vi "Realsense Cam Config Stream.vi"(8 "error in (no error)":errorcluster, 10 "Streams":T1[](array[typedef]), 11 "Realsense Cam in":refnum<class "Realsense Cam.lvclass">) -> (0 "error out":errorcluster, 3 "Realsense Cam out":refnum<class "Realsense Cam.lvclass">)   [LabVIEW 2018, in "Realsense Cam.lvclass"]
uses:
  Realsense Cam.lvclass
  Private/Stream Types Enum STYP.ctl
  Realsense Cam.lvclass/Realsense Cam.ctl
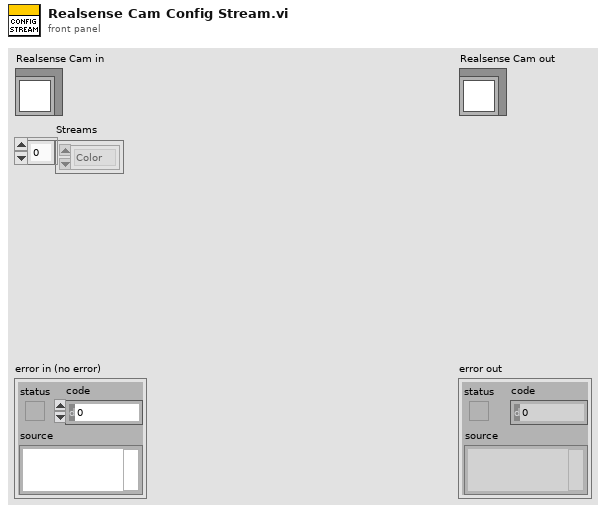
[diagram p1: front panel]
types:
  T1 = typedef "Realsense Cam.lvclass/Stream Types Enum STYP.ctl" = enum16{"Depth", "Left IR", "Right IR", "Color", "RGB Ext.", "Left IR Unrectified", "Right IR Unrectified"}
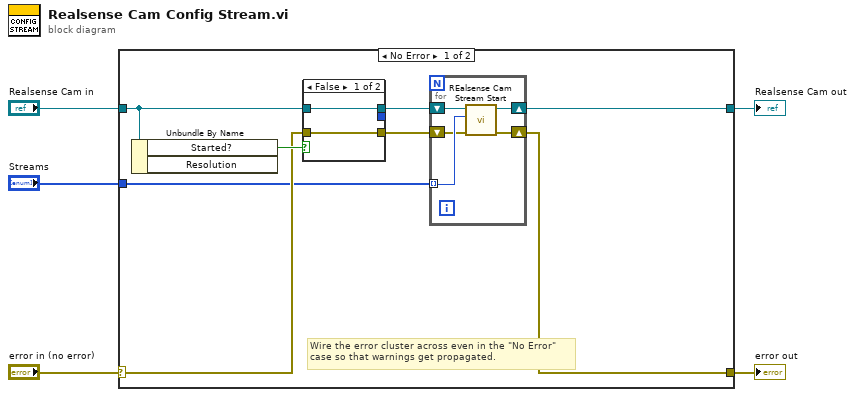
[diagram p0: block diagram]
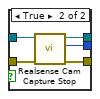
[diagram p2: hidden frame]
diagram:
  n1 = case shown="No Error" "error in (no error)" {
    selector: "error in (no error)" -> [w11 w27]
    tunnel: [w6 w27] -> w4
    tunnel: [w9 w26] -> w2
    tunnel: "Realsense Cam in" -> [w13 w26]
    tunnel: "Streams" -> [w8 _]
    frame No Error {
      # "Wire the error cluster across even in the \"No Error\"\ncase so that warnings get propagated."
      n2 = Unbundle By Name(w13) -> ("Started?"=w12:bool)  [unwired: 1 out]
      n3 = case shown="False" w12 {
        tunnel: w13 -> [w20 w25]
        tunnel: [w20 w22] -> w10
        tunnel: w11 -> [w19 w24]
        tunnel: [w19 w23] -> w7
        tunnel: [_ w21] -> _
        frame False {
        }
        frame True {
          n4 = call-dynamic "Realsense Cam Capture Stop.vi"("error in (no error)"=w24, "Realsense Cam in"=w25) -> ("error out"=w23:errorcluster, "error"=w21:u64, "Realsense Cam out"=w22:refnum<class "Realsense Cam.lvclass">)  [unwired: 7 in]
        }
      }
      n5 = for {
        shift-right: [w15] -> w9
        shift-left: w10 -> [w18]
        tunnel: w8 -> [w17] mode=indexing
        shift-right: [w14] -> w6
        shift-left: w7 -> [w16]
        n6 = call-dynamic "REalsense Cam Stream Start.vi"("error in (no error)"=w16, "Stream Type"=w17, "Realsense Cam in"=w18) -> ("error out"=w14:errorcluster, "Realsense Cam out"=w15:refnum<class "Realsense Cam.lvclass">)  [unwired: 7 in]
      }
    }
    frame Error {
    }
  }
  "error out" <- w4
  "Realsense Cam out" <- w2
